vi "HFRR ADV v016 new software.vi"() -> ()   [LabVIEW 2025] (continued)
                        n2565 = local write "EVENT LOG"(w3581) -> ()
                      }
                      frame #28 {
                        n2566 = Wait (ms)(milliseconds to wait=u32 50) -> ()  [unwired: 1 out]
                      }
                      frame #29 {
                        n2567 = local read "Set Rh"() -> (w3585:dbl)
                        n2568 = Number To Fractional String(number=w3585, precision (6)=i16 2) -> (F-format string=w3586:string)  [unwired: 2 in]
                        n2569 = Concatenate Strings("Set Humidity [%RH] :" ("Content"), w3586) -> (w3588:string)
                        n2570 = local read "EVENT LOG"() -> (w3590:string)
                        n2571 = call "Event Log.vi"("Content"=w3588, "EVENT LOG"=w3590) -> ("EVENT LOG"=w3589:string)  [unwired: 8 in, 1 out]
                        n2572 = local write "EVENT LOG"(w3589) -> ()
                      }
                      frame #30 {
                        n2573 = Wait (ms)(milliseconds to wait=u32 50) -> ()  [unwired: 1 out]
                      }
                      frame #31 {
                        n2574 = local read "test time"() -> (w3593:dbl)
                        n2575 = Number To Fractional String(number=w3593, precision (6)=i16 1) -> (F-format string=w3594:string)  [unwired: 2 in]
                        n2576 = Concatenate Strings("Test Duration [mins] :" ("Content"), w3594) -> (w3596:string)
                        n2577 = local read "EVENT LOG"() -> (w3598:string)
                        n2578 = call "Event Log.vi"("Content"=w3596, "EVENT LOG"=w3598) -> ("EVENT LOG"=w3597:string)  [unwired: 8 in, 1 out]
                        n2579 = local write "EVENT LOG"(w3597) -> ()
                      }
                      frame #32 {
                        w3599 = dbl[] [] ("History Data")
                        w3600 = cluster{"y":dbl, dbl, "y":dbl}[] [] ("History Data")
                        w3601 = FALSE ("Visible")
                        n2580 = property on="Stroke ( mm )" class="WFChart (strict)"("History Data"=w3600) -> ()  [unwired: 2 in, 2 out]
                        n2581 = property on="Humidity ( %RH )" class="WFChart (strict)"("History Data"=w3599) -> ()  [unwired: 2 in, 2 out]
                        n2582 = property on="Temperature ( Deg C )" class="WFChart (strict)"("History Data"=w3599) -> ()  [unwired: 2 in, 2 out]
                        n2583 = property on="Electrical Contact Resistance ( % )" class="WFChart (strict)"("History Data"=w3599) -> ()  [unwired: 2 in, 2 out]
                        n2584 = property on="Coefficient of Friction" class="WFChart (strict)"("History Data"=w3599) -> ()  [unwired: 2 in, 2 out]
                        n2585 = property on="Frictional Force ( N )" class="WFChart (strict)"("History Data"=w3599) -> ()  [unwired: 2 in, 2 out]
                        n2586 = property on="Coefficient of Friction" class="WFChart (strict)"("History Data"=w3599) -> ()  [unwired: 2 in, 2 out]
                        n2587 = property on="Frictional Force ( N )" class="WFChart (strict)"("History Data"=w3599) -> ()  [unwired: 2 in, 2 out]
                        n2588 = property on="Electrical Contact Resistance ( % )" class="WFChart (strict)"("History Data"=w3599) -> ()  [unwired: 2 in, 2 out]
                        n2589 = property on="Humidity ( %RH )" class="WFChart (strict)"("History Data"=w3599) -> ()  [unwired: 2 in, 2 out]
                        n2590 = property on="Stroke ( mm )" class="WFChart (strict)"("History Data"=w3600) -> ()  [unwired: 2 in, 2 out]
                        n2591 = property on="Temperature ( Deg C )" class="WFChart (strict)"("History Data"=w3599) -> ()  [unwired: 2 in, 2 out]
                        n2592 = property on="Service Password Log" class="Str"("Visible"=w3601) -> ()  [unwired: 2 in, 2 out]
                        n2593 = property on="Password 3" class="Clust (strict)"("Visible"=w3601) -> ()  [unwired: 2 in, 2 out]
                      }
                    }
                    "TEST FILE NAM,E SAVED" <- TRUE ("TEST FILE NAM,E SAVED")
                  }
                }
              }
            }
          }
        }
        n2594 = case shown="True" w2898 {
          frame False {
            n2595 = local write "tfalg"(0.0 ("tfalg")) -> ()
          }
          frame True {
            n2596 = local read "tfalg"() -> (w3043:dbl)
            n2597 = Equal?(x=w3043, y=0.0) -> (x = y?=w3044:bool)
            n2598 = case shown="True" w3044 {
              frame False {
              }
              frame True {
                n2599 = local read "Total No. of Tests"() -> (w3047:dbl)
                n2600 = local write "tfalg"(1.0 ("tfalg")) -> ()
                n2601 = local write "acq 2"(FALSE ("acq 2")) -> ()
                n2602 = Wait (ms)(milliseconds to wait=u32 200) -> ()  [unwired: 1 out]
                n2603 = Increment(x=w3047) -> (x+1=w3046:dbl)
                n2604 = local write "Total No. of Tests"(w3046) -> ()
              }
            }
          }
        }
        n2605 = local write "Test \nStatus"(w2904) -> ()
        n2606 = local write "Save"(w2904) -> ()
        n2607 = local read "Main Tab"() -> (w2861:T2)
        n2608 = case shown="True" w2885 {
          tunnel: [FALSE ("RUN") TRUE ("RUN")] -> w2884
          tunnel: [_ 1] -> w2877
          frame False {
          }
          frame True {
          }
        }
        n2609 = In Range and Coerce(upper limit=w2892, x=w2865, lower limit=w2891) -> (In Range?=w2883:bool)  [unwired: 1 out]
        n2610 = In Range and Coerce(upper limit=w2889, x=w2864, lower limit=w2890) -> (In Range?=w2881:bool)  [unwired: 1 out]
        n2611 = case shown="True" w2897 {
          frame False {
            n2612 = local read "Rt 3"() -> (w3025:bool)
            n2613 = case shown="True" w3025 {
              frame False {
              }
              frame True {
                n2614 = local write "Rt 3"(FALSE ("Rt 3")) -> ()
                n2615 = local write "Json End Flg"(TRUE ("Upld AR 2")) -> ()
              }
            }
            "Rt" <- TRUE ("Rt")
            "Rt 2" <- FALSE ("Rt")
          }
          frame True {
            n2616 = local read "Rt"() -> (w3032:bool)
            n2617 = local write "Rt 2"(TRUE ("Rt 2")) -> ()
            n2618 = case shown="True" w3032 {
              frame False {
              }
              frame True {
                w3033 = TRUE ("Upld AR 2")
                n2619 = local write "Rt"(FALSE ("Rt")) -> ()
                n2620 = local write "Upld AR"(w3033) -> ()
                n2621 = local write "Json St Flg"(w3033) -> ()
              }
            }
            "Rt 3" <- TRUE ("Rt 3")
          }
        }
        n2622 = case shown="True" w2883 {
          tunnel: [FALSE ("RUN") TRUE ("RUN")] -> w2882
          tunnel: [_ 2] -> w2876
          frame False {
          }
          frame True {
          }
        }
        n2623 = case shown="True" w2881 {
          tunnel: [FALSE ("RUN") TRUE ("RUN")] -> w2880
          tunnel: [_ 3] -> w2875
          frame False {
          }
          frame True {
          }
        }
        n2624 = case shown="\"Acquire\"" w2861 {
          tunnel: w2863 -> [_ w3094]
          frame Default {
            w3093 = 0.0 ("output")
            n2625 = local write "PID-out"(w3093) -> ()
            n2626 = local write "Frequency ( Hz )"(w3093) -> ()
          }
          frame "Acquire" {
            n2627 = stacked-sequence {
              frame #0 {
                n2628 = local read "Auto Start Test"() -> (w3096:bool)
                n2629 = case shown="True" w3096 {
                  tunnel: "RUN" -> [w3117 w3120]
                  tunnel: [w3117 w3119] -> w3097
                  frame False {
                  }
                  frame True {
                    n2630 = local read "Auto Start Temp"() -> (w3118:bool)
                    n2631 = Or(x=w3120, y=w3118) -> (x .or. y?=w3119:bool)
                  }
                }
                n2632 = local read "clk"() -> (w3116:dbl)
                n2633 = local read "Save"() -> (w3112:bool)
                n2634 = Equal?(x=w3116, y=0.0) -> (x = y?=w3113:bool)
                n2635 = And(x=w3113, y=w3112) -> (x .and. y?=w3114:bool)
                n2636 = Not(x="Engage") -> (.not. x?=w3103:bool)
                n2637 = case shown="False" w3097 {
                  tunnel: [0.0 w3143] -> w3099
                  frame False {
                    (unwired) TRUE ("Visible")
                    n2638 = local read "Auto Start Test"() -> (w3124:bool)
                    n2639 = local write "Start Time"(TRUE ("Start Time")) -> ()
                    n2640 = property on="Stroke 2" class="DigNum (strict)"("Visible"=FALSE) -> ()  [unwired: 2 in, 2 out]
                    n2641 = case shown="False" w3124 {
                      frame False {
                        n2642 = property on="Heater Button" class="Bool (strict)"("DisabledEnum"=T18."Enabled" ("Disabled")) -> ()  [unwired: 2 in, 2 out]
                        n2643 = property on="Humidity" class="Bool (strict)"("DisabledEnum"=T18."Enabled" ("Disabled")) -> ()  [unwired: 2 in, 2 out]
                      }
                      frame True {
                      }
                    }
                    n2644 = case shown="False" "TestCompFlg" {
                      frame False {
                        n2645 = local read "StartFlg"() -> (w3132:bool)
                        n2646 = case shown="True" w3132 {
                          frame False {
                          }
                          frame True {
                            n2647 = stacked-sequence {
                              frame #0 {
                                n2648 = local read "EVENT LOG"() -> (w3136:string)
                                n2649 = call "Event Log.vi"("Content"="Test was interrupted", "EVENT LOG"=w3136) -> ("EVENT LOG"=w3137:string)  [unwired: 8 in, 1 out]
                                n2650 = local write "EVENT LOG"(w3137) -> ()
                                n2651 = property on="RUN" class="Bool (strict)"("Visible"=TRUE) -> ()  [unwired: 2 in, 2 out]
                                n2652 = property on="Auto Start Test" class="Bool (strict)"("Visible"=TRUE) -> ()  [unwired: 2 in, 2 out]
                              }
                              frame #1 {
                                w3139 = FALSE ("StartFlg")
                                n2653 = property on="Heater Button" class="Bool (strict)"("Val(Sgnl)"=FALSE ("Value (Signaling)")) -> ()  [unwired: 2 in, 2 out]
                                n2654 = local write "Heater Button"(w3139) -> ()
                                n2655 = local write "StartFlg"(w3139) -> ()
                                n2656 = local write "Humidity"(w3139) -> ()
                              }
                              frame #2 {
                                n2657 = local write "Command"("VC;0" ("Command")) -> ()
                              }
                              frame #3 {
                                n2658 = Wait (ms)(milliseconds to wait=u32 1500) -> ()  [unwired: 1 out]
                              }
                              frame #4 {
                                n2659 = local write "Command"("HE;0" ("Command")) -> ()
                              }
                            }
                          }
                        }
                      }
                      frame True {
                      }
                    }
                    n2660 = local write "String 14"("Test will autostart once parameters reach the set value." ("String 14")) -> ()
                  }
                  frame True {
                    (unwired) FALSE ("Visible")
                    n2661 = property on="Stroke 2" class="DigNum (strict)"("Visible"=TRUE) -> ()  [unwired: 2 in, 2 out]
                    n2662 = property on="STOP 2" class="Bool (strict)"("Disabled"=u8 2) -> ()  [unwired: 2 in, 2 out]
                    n2663 = local write "String 14"(" Running....." ("String 14")) -> ()
                    n2664 = property on="Heater Button" class="Bool (strict)"("DisabledEnum"=T18."Disabled and Grayed Out" ("Disabled")) -> ()  [unwired: 2 in, 2 out]
                    n2665 = property on="Humidity" class="Bool (strict)"("DisabledEnum"=T18."Disabled and Grayed Out" ("Disabled")) -> ()  [unwired: 2 in, 2 out]
                    n2666 = case shown="True" "Start Time" {
                      selector: "Start Time" -> [_ w3162]
                      frame False {
                      }
                      frame True {
                        n2667 = Not(x=w3162) -> (.not. x?=w3161:bool)
                        n2668 = local write "Start Time"(w3161) -> ()
                        n2669 = local read "EVENT LOG"() -> (w3163:string)
                        n2670 = call "Event Log.vi"("Content"="Test in progress", "EVENT LOG"=w3163) -> ("EVENT LOG"=w3165:string)  [unwired: 8 in, 1 out]
                        n2671 = local write "EVENT LOG"(w3165) -> ()
                      }
                    }
                    n2672 = disable-structure shown="Enabled" {
                      disable-tunnel: [w3154 w3160] -> w3143
                      frame Disabled {
                        n2673 = local read "Set Hz"() -> (w3157:dbl)
                        n2674 = call <vilib>:"Uniform White Noise Waveform.vi"() -> ("signal out"=w3156:waveform(dbl))  [unwired: 10 in, 1 out]
                        n2675 = Random Number (0-1)() -> (number: 0 to 1=w3153:dbl)
                        n2676 = Add(x=w3157, y=w3156) -> (x+y=w3155:waveform(dbl))
                        n2677 = Multiply(x=ext 0.01 ("y"), y=w3153) -> (x*y=w3151:ext)
                        n2678 = Multiply(x=w3155, y=w3151) -> (x*y=w3154:waveform(ext))
                      }
                      frame Enabled {
                        n2679 = call-poly <vilib>:"Random Number (Range).vi"("lower bound (0)"=49.89, "upper bound (100)"=50.8) -> ("number"=w3160:dbl)  [unwired: 9 in]
                      }
                    }
                    "StartFlg" <- TRUE ("StartFlg")
                  }
                }
                n2680 = case shown="True" w3114 {
                  frame False {
                  }
                  frame True {
                    n2681 = local write "clk"(10.0 ("clk")) -> ()
                    n2682 = Get Date/Time In Seconds() -> (seconds since 1Jan1904=w3168:timestamp)
                    n2683 = To Double Precision Float(number=w3168) -> (double precision float=w3166:dbl)
                    n2684 = local write "acq timer"(w3166) -> ()
                    n2685 = local write "act save time"(w3166) -> ()
                  }
                }
                n2686 = call "Elapsed Time"("Time Target (s)"="Countdown", "Reset"=w3103) -> ("Elapsed Time (s)"=w3108:dbl, "Time has Elapsed"=w3106:bool)  [unwired: 10 in, 6 out]
                "Countdown 2" <- w3108
                n2687 = Subtract(x=w3108, y=2.0) -> (x-y=w3111:dbl)
                n2688 = Less?(x=w3111, y="Countdown") -> (x < y?=w3109:bool)
                n2689 = And(x=w3109, y=w3106) -> (x .and. y?=w3105:bool)
                n2690 = case shown="True" w3105 {
                  frame False {
                  }
                  frame True {
                    (unwired) dbl[] [] ("History Data")
                    n2691 = local write "Engage"(FALSE ("Engage")) -> ()
                    n2692 = local write "RUN"(TRUE ("RUN")) -> ()
                    n2693 = local read "Humidity ( %RH )"() -> (→"Rh Before":dbl)
                  }
                }
                n2694 = local read "Test \nStatus"() -> (w3101:bool)
                n2695 = Select(t=w3099, s=w3101, f=0.0) -> (s? t:f=w3100:dbl)
                n2696 = local write "Frequency ( Hz )"(w3100) -> ()
              }
              frame #1 {
                w3191 = 1000000.0 ("x")
                # "HC;1/0\nST;VALUE"
                # "Elapsed time\ncof\nstroke\nAir temp\nTemp\nHumidity"
                # "acq timer\n\nact save time"
                # "convert to microseconds"
                n2697 = local read "COUNT"() -> (w3174:i32)
                n2698 = local read "Rate"() -> (w3187:dbl)
                n2699 = Divide(x=w3191, y=w3187) -> (x/y=w3192:dbl)
                n2700 = Greater Or Equal?(x=w3174, y=250) -> (x >= y?=w3173:bool)
                n2701 = Get Date/Time In Seconds() -> (seconds since 1Jan1904=w3194:timestamp)
                n2702 = case shown="True" w3173 {
                  frame False {
                    n2703 = local read "COUNT"() -> (w3195:i32)
                    n2704 = Increment(x=w3195) -> (x+1=w3196:i32)
                    n2705 = local write "COUNT"(w3196) -> ()
                  }
                  frame True {
                    n2706 = local write "COUNT"(0 ("COUNT")) -> ()
                  }
                }
                n2707 = local read "Samplingtime 2"() -> (w3172:dbl)
                n2708 = local read "act save time"() -> (w3189:dbl)
                n2709 = Divide(x=w3192, y=w3191) -> (x/y=w3190:dbl)
                n2710 = To Double Precision Float(number=w3194) -> (double precision float=w3183:dbl)
                n2711 = Add(x=w3189, y=w3172) -> (x+y=w3188:dbl)
                n2712 = local read "acq timer"() -> (w3193:dbl)
                n2713 = local read "COUNT"() -> (w3176:i32)
                n2714 = Greater Or Equal?(x=w3183, y=w3188) -> (x >= y?=w3171:bool)
                n2715 = Multiply(x=w3190, y=w3176) -> (x*y=w3182:dbl)
                n2716 = Subtract(x=w3183, y=w3193) -> (x-y=w3185:dbl)
                n2717 = local read "Save"() -> (w3186:bool)
                n2718 = Add(x=w3185, y=w3182) -> (x+y=w3169:dbl)
                "Elapsed time 3" <- w3169
                n2719 = And(x=w3171, y=w3186) -> (x .and. y?=w3184:bool)
                n2720 = Divide(x=w3169, y=60.0) -> (x/y=w3180:dbl)
                n2721 = local read "Test \nStatus"() -> (w3170:bool)
                n2722 = local read "clk"() -> (w3177:dbl)
                n2723 = Equal?(x=w3177, y=10.0) -> (x = y?=w3179:bool)
                n2724 = case shown="True" w3184 {
                  tunnel: w3183 -> [_ w3307]
                  tunnel: [FALSE ("Boolean 2") TRUE ("Boolean 2")] -> _
                  frame False {
                  }
                  frame True {
                    w3261 = ";" ("Substring")
                    # "Pid out/\nFreq response value"
                    n2725 = local write "act save time"(w3307) -> ()
                    n2726 = local read "FILE"() -> (w3255:string)
                    n2727 = call "file check.vi"("file name in"=w3255) -> ("error out"=w3258:errorcluster, "file name out"=w3253:string)  [unwired: 9 in]
                    n2728 = local read "LVDT STROKE"() -> (w3250:dbl)
                    n2729 = local read "Add up Stroke"() -> (w3248:dbl)
                    n2730 = call "FILE PATH CREATION.vi"("error in"=w3258, "FILE NAME :"=w3253) -> ("FILE OUT"=w3256:path)  [unwired: 8 in, 1 out]
                    n2731 = Concatenate Strings(w3253, ".dgf" ("Substring")) -> (w3257:string)
                    n2732 = Subtract(x=w3250, y=w3248) -> (x-y=w3249:dbl)
                    n2733 = Absolute Value(x=w3249) -> (abs(x)=w3247:dbl)
                    n2734 = local read "FF 2"() -> (→"Frictional Force ( N )" →"Frictional Force ( N )":dbl)
                    n2735 = Build Path(base path=w3256, name or relative path=w3257) -> (appended path=w3252:path)
                    n2736 = local read "COF 2"() -> (w3266:dbl)
                    "cof" <- w3266
                    "Coefficient of Friction" <- w3266
                    "COF 4" <- w3266
                    "Coefficient of Friction" <- w3266
                    n2737 = local read "TEMP"() -> (w3269:dbl)
                    "Temp" <- w3269
                    "Temperature ( Deg C )" <- w3269
                    n2738 = local read "Humidity ( %RH )"() -> (w3268:dbl)
                    "Humidity ( %RH )" <- w3268
                    "Humidity ( %RH )" <- w3268
                    n2739 = local read "Frequency ( Hz )"() -> (w3275:dbl)
                    n2740 = call <vilib>:"Mean PtByPt.vi"("x"=w3247, "sample length"="STROKE FILTER") -> ("mean"=w3246:dbl)  [unwired: 2 in, 1 out]
                    n2741 = local read "Elapsed time"() -> (w3300:dbl)
                    n2742 = local read "AIR TEMP"() -> (w3273:dbl)
                    n2743 = local read "PID-out"() -> (w3278:dbl)
                    n2744 = local write "Temperature ( Deg C )"(w3269) -> ()
                    n2745 = Number To Fractional String(number=w3246, width (-)=i16 9 ("precision (6)"), precision (6)=i16 6) -> (F-format string=w3293:string)  [unwired: 1 in]
                    n2746 = Number To Fractional String(number=w3273, width (-)=i16 9 ("precision (6)"), precision (6)=i16 3) -> (F-format string=w3292:string)  [unwired: 1 in]
                    n2747 = Number To Fractional String(number=w3269, width (-)=i16 9 ("precision (6)"), precision (6)=i16 3) -> (F-format string=w3289:string)  [unwired: 1 in]
                    n2748 = Number To Fractional String(number=w3268, width (-)=i16 9 ("precision (6)"), precision (6)=i16 3) -> (F-format string=w3286:string)  [unwired: 1 in]
                    n2749 = Number To Fractional String(number=0.0, width (-)=i16 9 ("precision (6)"), precision (6)=i16 3) -> (F-format string=w3283:string)  [unwired: 1 in]
                    n2750 = Number To Fractional String(number=w3278, width (-)=i16 9 ("precision (6)"), precision (6)=i16 3) -> (F-format string=w3279:string)  [unwired: 1 in]
                    n2751 = Number To Fractional String(number=w3275, width (-)=i16 9 ("precision (6)"), precision (6)=i16 3) -> (F-format string=w3274:string)  [unwired: 1 in]
                    n2752 = Number To Fractional String(number=w3266, width (-)=i16 9 ("precision (6)"), precision (6)=i16 6) -> (F-format string=w3301:string)  [unwired: 1 in]
                    n2753 = Number To Fractional String(number=w3300, width (-)=i16 14 ("precision (6)"), precision (6)=i16 3) -> (F-format string=w3302:string)  [unwired: 1 in]
                    n2754 = Bundle("y"=1.02, "mean"=w3246, "y"=0.98) -> (w3267:cluster{"y":dbl, "mean":dbl, "y":dbl})  [unwired: 1 in]
                    n2755 = Number To Fractional String(number="Ambient Humidity :", width (-)=i16 9 ("precision (6)"), precision (6)=i16 6) -> (F-format string=w3259:string)  [unwired: 1 in]
                    n2756 = local read "RUN"() -> (w3265:bool)
                    n2757 = case shown="True" w3265 {
                      tunnel: w3267 -> [_ w3312]
                      tunnel: w3246 -> [_ w3311]
                      tunnel: w3246 -> [_ w3309]
                      tunnel: w3246 -> [_ w3310]
                      frame False {
                      }
                      frame True {
                        "Stroke ( mm )" <- w3312
                        "Stroke ( mm )" <- w3312
                        "Stroke 4" <- w3311
                        "Stroke 3" <- w3309
                        "Stroke 2" <- w3310
                        "measured_stroke" <- w3309
                      }
                    }
                    n2758 = Concatenate Strings(w3302, w3261, w3301, w3261, w3293, w3261, w3292, w3261, w3289, w3261, w3286, w3261, w3283, w3261, w3279, w3261, w3274, w3261, w3259, "\r") -> (w3299:string)
                    n2759 = call <vilib>:"Write Characters To File.vi"("append to file? (new file:F)"=TRUE, "character string"=w3299, "file path (dialog if empty)"=w3252) -> ()  [unwired: 2 in, 1 out]
                    "refresh flag" <- TRUE ("refresh flag")
                  }
                }
                n2760 = case shown="True" w3170 {
                  tunnel: w3180 -> [_ w3206]
                  tunnel: w3185 -> [_ w3216]
                  tunnel: [0.0 w3212] -> _
                  tunnel: w3179 -> [_ w3211]
                  tunnel: [0.0 w3210] -> _
                  tunnel: w3169 -> [_ w3210]
                  tunnel: w3183 -> [w3199 _]
                  frame False {
                    n2761 = local write "acq timer"(w3199) -> ()
                    n2762 = local write "Test Duration Status"(0.0 ("Test Duration Status")) -> ()
                  }
                  frame True {
                    n2763 = local read "Set Hz"() -> (w3213:dbl)
                    n2764 = local write "Elapsed time"(w3206) -> ()
                    n2765 = local read "test time"() -> (w3205:dbl)
                    n2766 = Multiply(x=w3216, y=w3213) -> (x*y=w3215:dbl)
                    n2767 = case shown="False" w3211 {
                      tunnel: w3215 -> [w3217 _]
                      tunnel: [w3217 1.0] -> w3212
                      frame False {
                        n2768 = local write "Cycles elapsed"(w3217) -> ()
                      }
                      frame True {
                      }
                    }
                    n2769 = Greater?(x=w3206, y=w3205) -> (0:w3214:bool)
                    n2770 = Subtract(x=w3205, y=w3206) -> (x-y=w3204:dbl)
                    "time" <- w3204
                    n2771 = Multiply(x=w3204, y=60.0) -> (x*y=w3203:dbl)
                    n2772 = local write "Time Remaining"(w3203) -> ()
                    n2773 = local write "Remaining Time"(w3203) -> ()
                    n2774 = case shown="True" w3214 {
                      frame False {
                      }
                      frame True {
                        n2775 = stacked-sequence {
                          frame #0 {
                            w3222 = T18."Enabled" ("Disabled")
                            w3221 = FALSE ("TEST FILE NAM,E SAVED")
                            w3223 = "" ("FILE")
                            w3224 = TRUE ("Visible")
                            n2776 = local write "Humidity"(FALSE ("Humidity")) -> ()
                            n2777 = local write "RUN"(FALSE ("OK Button 2")) -> ()
                            n2778 = local write "Heater Button"(FALSE ("Heater Button")) -> ()
                            n2779 = local write "Auto Start Test"(FALSE ("Auto Start Test")) -> ()
                            n2780 = local write "TestCompFlg"(TRUE ("StpFlg")) -> ()
                            n2781 = local read "Humidity ( %RH )"() -> (→"Rh After":dbl)
                            n2782 = property on="STOP 2" class="Bool (strict)"("Disabled"=u8 0) -> ()  [unwired: 2 in, 2 out]
                            n2783 = local read "EVENT LOG"() -> (w3229:string)
                            n2784 = call "Event Log.vi"("Content"="Test Completed", "EVENT LOG"=w3229) -> ("EVENT LOG"=w3228:string)  [unwired: 8 in, 1 out]
                            n2785 = property on="RUN" class="Bool (strict)"("Visible"=w3224) -> ()  [unwired: 2 in, 2 out]
                            n2786 = property on="Auto Start Test" class="Bool (strict)"("Visible"=w3224) -> ()  [unwired: 2 in, 2 out]
                            n2787 = local write "Batch Ref Num :"(w3223) -> ()
                            n2788 = local write "FILE"(w3223) -> ()
                            n2789 = local write "EVENT LOG"(w3228) -> ()
                            n2790 = local write "TEST FILE NAM,E SAVED"(w3221) -> ()
                            n2791 = local write "Fuel Discription :"(w3223) -> ()
                            n2792 = local write "START TEMP"(w3221) -> ()
                            n2793 = local write "Remarks :"(w3223) -> ()
                            n2794 = local write "Main Dashboard Buttons"(T1."Imaging" ("Main Dashboard Buttons")) -> ()
                            n2795 = local write "Main Tab"(T2."Adv Scar" ("Main Tab")) -> ()
                            n2796 = property on="FRICVALZ 2" class="Bool (strict)"("DisabledEnum"=w3222) -> ()  [unwired: 2 in, 2 out]
                            n2797 = property on="FRICVALZ 3" class="Bool (strict)"("DisabledEnum"=w3222) -> ()  [unwired: 2 in, 2 out]
                            n2798 = property on="FRICVALZ 4" class="Bool (strict)"("DisabledEnum"=w3222) -> ()  [unwired: 2 in, 2 out]
                          }
                          frame #1 {
                            n2799 = Wait (ms)(milliseconds to wait=u32 1500) -> ()  [unwired: 1 out]
                          }
                          frame #2 {
                            n2800 = local write "Command"("VC;0") -> ()
                          }
                          frame #3 {
                            n2801 = Wait (ms)(milliseconds to wait=u32 1500) -> ()  [unwired: 1 out]
                          }
                          frame #4 {
                            n2802 = local write "Command"("VC;0") -> ()
                          }
                          frame #5 {
                            n2803 = Wait (ms)(milliseconds to wait=u32 1500) -> ()  [unwired: 1 out]
                          }
                          frame #6 {
                            n2804 = local write "Command"("ST;0") -> ()
                          }
                          frame #7 {
                            n2805 = local write "measured_stroke"(0.0 ("measured_stroke")) -> ()
                            n2806 = Wait (ms)(milliseconds to wait=u32 1500) -> ()  [unwired: 1 out]
                          }
                          frame #8 {
                            n2807 = local write "Command"("HE;0") -> ()
                          }
                        }
                      }
                    }
                    n2808 = Divide(x=w3206, y=w3205) -> (x/y=w3209:dbl)
                    n2809 = Multiply(x=w3209, y=100.0) -> (x*y=w3207:dbl)
                    n2810 = local write "Test Duration Status"(w3207) -> ()
                  }
                }
              }
              frame #2 {
                n2811 = case shown="True" "Heater Button" {
                  tunnel: [0.0 ("output") w3335] -> w3313
                  frame False {
                    w3316 = TRUE ("tmpchk")
                    n2812 = local read "TEMP"() -> (w3317:dbl)
                    n2813 = local write "Temp ini"(w3317) -> ()
                    n2814 = local write "Reset 4"(w3316) -> ()
                    n2815 = local write "tmpchk"(w3316) -> ()
                    n2816 = local write "reinit"(TRUE ("reinit")) -> ()
                    n2817 = local write "manual temp log"(TRUE ("manual temp log")) -> ()
                  }
                  frame True {
                    # "Logic to turn off\nthe heater when \ntemp is not rising.\nTime - 60 sec\nDelta t- 5°c"
                    n2818 = local read "Temp ini"() -> (w3324:dbl)
                    n2819 = local read "Auto Start Test"() -> (w3320:bool)
                    n2820 = Less?(x=w3324, y=53.0) -> (x < y?=w3322:bool)
                    n2821 = case shown="False" w3320 {
                      frame False {
                        n2822 = local read "Set Temp"() -> (w3344:dbl)
                        n2823 = local read "TEMP"() -> (w3343:dbl)
                        n2824 = Subtract(x=w3344, y=w3343) -> (x-y=w3342:dbl)
                        n2825 = Absolute Value(x=w3342) -> (abs(x)=w3341:dbl)
                        n2826 = Less?(x=w3341, y=0.5) -> (x < y?=w3339:bool)
                        n2827 = case shown="True" w3339 {
                          tunnel: "manual temp log" -> [_ w3345]
                          frame False {
                          }
                          frame True {
                            n2828 = case shown="True" w3345 {
                              selector: w3345 -> [_ w3346]
                              frame False {
                              }
                              frame True {
                                # "#Event log"
                                n2829 = Not(x=w3346) -> (.not. x?=w3347:bool)
                                n2830 = local write "manual temp log"(w3347) -> ()
                                n2831 = local read "EVENT LOG"() -> (w3350:string)
                                n2832 = call "Event Log.vi"("Content"="Target Temperature reached", "EVENT LOG"=w3350) -> ("EVENT LOG"=w3349:string)  [unwired: 8 in, 1 out]
                                n2833 = local write "EVENT LOG"(w3349) -> ()
                              }
                            }
                          }
                        }
                      }
                      frame True {
                        n2834 = local write "manual temp log"(TRUE ("manual temp log")) -> ()
                      }
                    }
                    n2835 = And(x="tmpchk", y=w3322) -> (x .and. y?=w3325:bool)
                    n2836 = case shown="True" w3325 {
                      frame False {
                      }
                      frame True {
                        n2837 = call "Elapsed Time8"("Time Target (s)"=300.0, "Reset"="Reset 4") -> ("Time has Elapsed"=w3352:bool)  [unwired: 10 in, 7 out]
                        n2838 = flat-sequence {
                          tunnel: w3352 -> [_]
                          frame #0 {
                            n2839 = local write "Reset 4"(FALSE ("Reset 4")) -> ()
                          }
                        }
                        n2840 = case shown="True" w3352 {
                          frame False {
                          }
                          frame True {
                            n2841 = local read "Temp ini"() -> (w3359:dbl)
                            n2842 = Add(x=w3359, y=5.0) -> (x+y=w3357:dbl)
                            n2843 = local read "TEMP"() -> (w3360:dbl)
                            n2844 = Greater?(x=w3360, y=w3357) -> (0:w3358:bool)
                            n2845 = case shown="False" w3358 {
                              frame False {
                                n2846 = local write "Heater Button"(FALSE ("Heater Button")) -> ()
                              }
                              frame True {
                                n2847 = local write "tmpchk"(FALSE ("tmpchk")) -> ()
                              }
                            }
                          }
                        }
                      }
                    }
                    n2848 = local read "Set Temp"() -> (w3333:dbl)
                    n2849 = local read "TEMP"() -> (w3327:dbl)
                    n2850 = call-poly <vilib>:"PID.vi"("reinitialize? (F)"="reinit", "dt (s)"=-1.0, "process variable"=w3327, "setpoint"=w3333) -> ("output"=w3330:dbl)  [unwired: 6 in, 1 out]
                    n2851 = Subtract(x=w3333, y=w3327) -> (x-y=w3334:dbl)
                    n2852 = Add(x=w3333, y=0.5) -> (x+y=w3331:dbl)
                    n2853 = Greater Or Equal?(x=w3327, y=w3331) -> ()  [unwired: 1 out]
                    n2854 = Select(t=0.0, s=FALSE, f=w3330) -> (s? t:f=w3329:dbl)
                    "PID output" <- w3329
                    n2855 = flat-sequence {
                      tunnel: w3329 -> [w3363]
                      tunnel: [w3363] -> w3335
                      frame #0 {
                        n2856 = local write "reinit"(FALSE ("reinit")) -> ()
                      }
                    }
                    n2857 = Bundle(w3334, "output"=w3329, "TEMP"=w3327) -> ()  [unwired: 1 in, 1 out]
                  }
                }
                "PID-out" <- w3313
              }
              frame #3 {
                n2858 = local read "TEMP"() -> (w3365:dbl)
                n2859 = Greater Or Equal?(x=w3365, y="Set Temp 2") -> (x >= y?=w3370:bool)
                n2860 = case shown="True" w3370 {
                  tunnel: [FALSE TRUE] -> w3368
                  frame False {
                  }
                  frame True {
                  }
                }
                "Status 13" <- w3368
                n2861 = And(x=w3368, y="trip1 8") -> (x .and. y?=w3367:bool)
                n2862 = case shown="True" w3367 {
                  frame False {
                    n2863 = local write "Heater Trip Temp"(TRUE ("Heater Trip Temp")) -> ()
                  }
                  frame True {
                    w3373 = FALSE ("OK Button 2")
                    n2864 = case shown="True" "Heater Trip Temp" {
                      selector: "Heater Trip Temp" -> [_ w3375]
                      frame False {
                      }
                      frame True {
                        n2865 = Not(x=w3375) -> (.not. x?=w3374:bool)
                        n2866 = local read "EVENT LOG"() -> (w3378:string)
                        n2867 = local write "Heater Trip Temp"(w3374) -> ()
                        n2868 = call "Event Log.vi"("Content"="Heater Trip", "EVENT LOG"=w3378) -> ("EVENT LOG"=w3377:string)  [unwired: 8 in, 1 out]
                        n2869 = local write "EVENT LOG"(w3377) -> ()
                      }
                    }
                    n2870 = local write "RUN"(w3373) -> ()
                    n2871 = property on="Auto Start Test" class="Bool (strict)"("Value"=w3373) -> ()  [unwired: 2 in, 2 out]
                    n2872 = local write "Heater Button"(w3373) -> ()
                  }
                }
              }
            }
            n2873 = case shown="False" w3094 {
              frame False {
                n2874 = disable-structure shown="Disabled" {
                  frame Disabled {
                    n2875 = stacked-sequence {
                      frame #0 {
                        n2876 = local write "RUN"(FALSE ("OK Button 2")) -> ()
                      }
                      frame #1 {
                      }
                    }
                  }
                  frame Enabled {
                  }
                }
              }
              frame True {
              }
            }
          }
        }
        n2877 = local read "airtempflg"() -> (w2886:bool)
        n2878 = Or(x=w2886, y=w2884) -> (x .or. y?=w2887:bool)
        n2879 = Insert Into Array(array=string[] ["Air Temperature has reached set value,", "Humidity has reached set value,", "Sample Temperaturehas reached set value,", ""], index=0, new element="") -> (w2872:string[])
        n2880 = Build Array(w2877, w2876, w2875) -> (w2873:i32[])
        n2881 = disable-structure shown="Disabled" {
          disable-tunnel: w2887 -> [w2964 _]
          disable-tunnel: w2882 -> [w2963 _]
          disable-tunnel: w2880 -> [w2962 _]
          frame Disabled {
            n2882 = Compound Arithmetic op=AND(w2964, w2963, w2962) -> ()  [unwired: 1 out]
            n2883 = case shown="True" {
              selector: _ -> [_ _]
              frame False {
              }
              frame True {
                w2965 = FALSE ("autostrtflg")
                n2884 = local write "RUN"(TRUE ("RUN")) -> ()
                n2885 = local write "autostrtflg"(w2965) -> ()
                n2886 = local write "autostart"(w2965) -> ()
                n2887 = local write "String 14"(" Running....." ("String 14")) -> ()
              }
            }
          }
          frame Enabled {
          }
        }
        n2888 = for {
          tunnel: w2873 -> [w3015] mode=indexing
          tunnel: w2872 -> [w3014]
          shift-right: [w3011] -> w2871
          shift-left: "" -> [w3013]
          n2889 = Index Array(array=w3014, index=w3015) -> (element=w3012:string)
          n2890 = Concatenate Strings(w3012, w3013) -> (w3011:string)
        }
        n2891 = local write "autostart 2"(w2871) -> ()
        n2892 = local read "Reset Graph"() -> (w2860:bool)
        n2893 = case shown="True" w2860 {
          selector: w2860 -> [_ w2914]
          frame False {
          }
          frame True {
            w2928 = 0.0 ("X Scale.Range:Maximum")
            n2894 = Not(x=w2914) -> (.not. x?=w2913:bool)
            n2895 = local write "Reset Graph"(w2913) -> ()
            n2896 = property on="Electrical Contact Resistance ( % )" class="WFChart (strict)"("XScale.Maximum"=600.0 ("X Scale.Range:Maximum"), "XScale.Minimum"=0.0 ("X Scale.Range:Minimum"), "YScale.Maximum"=100.0 ("Y Scale.Range:Maximum"), "YScale.Minimum"=0.0 ("Y Scale.Range:Minimum")) -> ()  [unwired: 2 in, 2 out]
            n2897 = property on="Frictional Force ( N )" class="WFChart (strict)"("XScale.Maximum"=600.0 ("X Scale.Range:Maximum"), "XScale.Minimum"=0.0 ("X Scale.Range:Minimum"), "YScale.Maximum"=100.0 ("Y Scale.Range:Maximum"), "YScale.Minimum"=0.0 ("Y Scale.Range:Minimum")) -> ()  [unwired: 2 in, 2 out]
            n2898 = property on="Temperature ( Deg C )" class="WFChart (strict)"("XScale.Maximum"=600.0 ("X Scale.Range:Maximum"), "XScale.Minimum"=0.0 ("X Scale.Range:Minimum"), "YScale.Maximum"=100.0 ("Y Scale.Range:Maximum"), "YScale.Minimum"=0.0 ("Y Scale.Range:Minimum")) -> ()  [unwired: 2 in, 2 out]
            n2899 = property on="Humidity ( %RH )" class="WFChart (strict)"("XScale.Maximum"=600.0 ("X Scale.Range:Maximum"), "XScale.Minimum"=0.0 ("X Scale.Range:Minimum"), "YScale.Maximum"=100.0 ("Y Scale.Range:Maximum"), "YScale.Minimum"=0.0 ("Y Scale.Range:Minimum")) -> ()  [unwired: 2 in, 2 out]
            n2900 = property on="Stroke ( mm )" class="WFChart (strict)"("XScale.Maximum"=600.0 ("X Scale.Range:Maximum"), "XScale.Minimum"=0.0 ("X Scale.Range:Minimum"), "YScale.Maximum"=100.0 ("Y Scale.Range:Maximum"), "YScale.Minimum"=0.0 ("Y Scale.Range:Minimum")) -> ()  [unwired: 2 in, 2 out]
            n2901 = property on="Coefficient of Friction" class="WFChart (strict)"("XScale.Maximum"=600.0 ("X Scale.Range:Maximum"), "XScale.Minimum"=0.0 ("X Scale.Range:Minimum"), "YScale.Maximum"=100.0 ("Y Scale.Range:Maximum"), "YScale.Minimum"=0.0 ("Y Scale.Range:Minimum")) -> ()  [unwired: 2 in, 2 out]
            n2902 = property on="Electrical Contact Resistance ( % )" class="WFChart (strict)"("XScale.Minimum"=0.0 ("X Scale.Range:Minimum"), "XScale.Maximum"=600.0 ("X Scale.Range:Maximum"), "YScale.Minimum"=0.0 ("Y Scale.Range:Minimum"), "YScale.Maximum"=100.0 ("Y Scale.Range:Maximum")) -> ()  [unwired: 2 in, 2 out]
            n2903 = property on="Temperature ( Deg C )" class="WFChart (strict)"("XScale.Minimum"=0.0 ("X Scale.Range:Minimum"), "XScale.Maximum"=600.0 ("X Scale.Range:Maximum"), "YScale.Minimum"=0.0 ("Y Scale.Range:Minimum"), "YScale.Maximum"=100.0 ("Y Scale.Range:Maximum")) -> ()  [unwired: 2 in, 2 out]
            n2904 = property on="Coefficient of Friction" class="WFChart (strict)"("XScale.Minimum"=0.0 ("X Scale.Range:Minimum"), "XScale.Maximum"=600.0 ("X Scale.Range:Maximum"), "YScale.Maximum"=1.0 ("X Scale.Range:Minimum"), "YScale.Minimum"=0.0 ("X Scale.Range:Minimum")) -> ()  [unwired: 2 in, 2 out]
            n2905 = property on="Frictional Force ( N )" class="WFChart (strict)"("XScale.Maximum"=600.0 ("X Scale.Range:Maximum"), "XScale.Minimum"=w2928, "YScale.Maximum"=10.0 ("Y Scale.Range:Maximum"), "YScale.Minimum"=w2928) -> ()  [unwired: 2 in, 2 out]
            n2906 = property on="Stroke ( mm )" class="WFChart (strict)"("XScale.Maximum"=600.0 ("X Scale.Range:Maximum"), "XScale.Minimum"=0.0 ("X Scale.Range:Minimum"), "YScale.Maximum"=100.0 ("Y Scale.Range:Maximum"), "YScale.Minimum"=0.0 ("Y Scale.Range:Minimum")) -> ()  [unwired: 2 in, 2 out]
            n2907 = property on="Humidity ( %RH )" class="WFChart (strict)"("XScale.Maximum"=600.0 ("X Scale.Range:Maximum"), "XScale.Minimum"=0.0 ("X Scale.Range:Minimum"), "YScale.Maximum"=100.0 ("Y Scale.Range:Maximum"), "YScale.Minimum"=0.0 ("Y Scale.Range:Minimum")) -> ()  [unwired: 2 in, 2 out]
          }
        }
      }
      frame "Compare Files" {
        # "Elapsed time\ncof\nstroke\nAir temp\nTemp\nHumidity"
        n2908 = case shown="True" "RSTV1 2" {
          frame False {
          }
          frame True {
            n2909 = property on="Humidity ( %RH )" class="XYGraph (strict)"("Y Scale.Display Format:Precision"=u8 0 ("Y Scale.Format & Precision:Precision")) -> ()  [unwired: 2 in, 2 out]
            n2910 = property on="Humidity ( %RH )" class="XYGraph (strict)"("X Scale.Range:Minimum"=0.0, "X Scale.Range:Maximum"=75.0, "Y Scale.Range:Minimum"=48.0, "Y Scale.Range:Maximum"=58.0) -> ()  [unwired: 2 in, 2 out]
          }
        }
        n2911 = case shown="True" "RST CP 2" {
          frame False {
          }
          frame True {
            n2912 = property on="XY Graph 13" class="XYGraph (strict)"("Y Scale.Display Format:Precision"=u8 0 ("Y Scale.Format & Precision:Precision")) -> ()  [unwired: 2 in, 2 out]
            n2913 = property on="XY Graph 13" class="XYGraph (strict)"("X Scale.Range:Minimum"=0.0, "X Scale.Range:Maximum"=75.0, "Y Scale.Range:Minimum"=0.0, "Y Scale.Range:Maximum"=100.0) -> ()  [unwired: 2 in, 2 out]
          }
        }
        n2914 = case shown="True" "RST CP" {
          frame False {
          }
          frame True {
            n2915 = property on="Sample Temperature ( °C )" class="XYGraph (strict)"("Y Scale.Display Format:Precision"=u8 2 ("Y Scale.Format & Precision:Precision")) -> ()  [unwired: 2 in, 2 out]
            n2916 = property on="Sample Temperature ( °C )" class="XYGraph (strict)"("X Scale.Range:Minimum"=0.0, "X Scale.Range:Maximum"=75.0, "Y Scale.Range:Minimum"=58.0, "Y Scale.Range:Maximum"=62.0) -> ()  [unwired: 2 in, 2 out]
          }
        }
        n2917 = case shown="True" "RSTV1 3" {
          frame False {
          }
          frame True {
            n2918 = property on="Air Temperature  ( °C )" class="XYGraph (strict)"("Y Scale.Display Format:Precision"=u8 2 ("Y Scale.Format & Precision:Precision")) -> ()  [unwired: 2 in, 2 out]
            n2919 = property on="Air Temperature  ( °C )" class="XYGraph (strict)"("X Scale.Range:Minimum"=0.0 ("Y Scale.Range:Minimum"), "X Scale.Range:Maximum"=75.0 ("Y Scale.Range:Maximum"), "Y Scale.Range:Minimum"=20.0 ("X Scale.Range:Minimum"), "Y Scale.Range:Maximum"=26.0 ("X Scale.Range:Maximum")) -> ()  [unwired: 2 in, 2 out]
          }
        }
        n2920 = case shown="True" "RSTV1 4" {
          frame False {
          }
          frame True {
            n2921 = property on="Stroke ( mm )" class="XYGraph (strict)"("Y Scale.Display Format:Precision"=u8 2 ("Y Scale.Format & Precision:Precision")) -> ()  [unwired: 2 in, 2 out]
            n2922 = property on="Stroke ( mm )" class="XYGraph (strict)"("X Scale.Range:Minimum"=0.0 ("Y Scale.Range:Maximum"), "X Scale.Range:Maximum"=75.0 ("X Scale.Range:Minimum"), "Y Scale.Range:Minimum"=0.98, "Y Scale.Range:Maximum"=1.02) -> ()  [unwired: 2 in, 2 out]
          }
        }
        n2923 = case shown="True" "rstv2" {
          frame False {
          }
          frame True {
            n2924 = property on="Coefficient Of Friction" class="XYGraph (strict)"("Y Scale.Display Format:Precision"=u8 3 ("Y Scale.Format & Precision:Precision")) -> ()  [unwired: 2 in, 2 out]
            n2925 = property on="Coefficient Of Friction" class="XYGraph (strict)"("X Scale.Range:Minimum"=0.0 ("Y Scale.Range:Maximum"), "X Scale.Range:Maximum"=75.0, "Y Scale.Range:Minimum"=0.0, "Y Scale.Range:Maximum"=1.0 ("X Scale.Range:Minimum")) -> ()  [unwired: 2 in, 2 out]
          }
        }
        n2926 = case shown="True" "RST CP 3" {
          frame False {
          }
          frame True {
            n2927 = property on="Air Temp ( °C ) vs Humidity ( % RH )" class="XYGraph (strict)"("X Scale.Range:Minimum"=18.0, "X Scale.Range:Maximum"=28.0 ("X Scale.Range:Minimum"), "Y Scale.Range:Minimum"=30.0 ("X Scale.Range:Minimum"), "Y Scale.Range:Maximum"=70.0 ("X Scale.Range:Minimum")) -> ()  [unwired: 2 in, 2 out]
          }
        }
        n2928 = case shown="True" "OPEN 1" {
          frame False {
          }
          frame True {
            (unwired) 0  # existing file
            w3654 = "Choose a datalog file to open"  # prompt
            n2929 = local write "OPEN 1"(FALSE ("OPEN 1")) -> ()
            n2930 = String To Path(string="C:\\LAB-IQ\\Data\\") -> (path=w3639:path)
            n2931 = File Dialog(6:"*.dgf" ("pattern"), 7:w3654, 11:w3639) -> (0:w3637:errorcluster, 3:w3645:path)  [unwired: 4 in, 2 out]
            n2932 = Unbundle(w3637) -> ()  [unwired: 3 out]
            n2933 = Strip Path(path=w3645) -> (name=w3644:string)  [unwired: 1 out]
            n2934 = Path To String(path=w3645) -> (string=w3640:string)
            "string1" <- w3640
            n2935 = Match Pattern(string=w3644, regular expression=".dgf") -> (before substring=→"String Control":string)  [unwired: 1 in, 3 out]
            n2936 = Match Pattern(string=w3640, regular expression=".dgf" ("substring (\"\")")) -> (before substring=w3650:string)  [unwired: 1 in, 3 out]
            n2937 = Concatenate Strings(w3650, ".duf" ("Substring")) -> (w3646:string)
            n2938 = String To Path(string=w3646) -> (path=w3651:path)
            n2939 = call <vilib>:"Read Characters From File.vi"("file path (dialog if empty)"=w3651, "start of read offset (chars.:0)"=60 ("start of read offset (chars.: 0)")) -> ("character string"=→"String Control 2":string)  [unwired: 4 in, 3 out]
          }
        }
        n2940 = case shown="True" "OPEN 2" {
          frame False {
          }
          frame True {
            (unwired) 0  # existing file
            w3672 = "Choose a datalog file to open"  # prompt
            n2941 = local write "OPEN 2"(FALSE ("OPEN 1")) -> ()
            n2942 = String To Path(string="C:\\LAB-IQ\\Data\\") -> (path=w3657:path)
            n2943 = File Dialog(6:"*.dgf" ("pattern"), 7:w3672, 11:w3657) -> (0:w3655:errorcluster, 3:w3663:path)  [unwired: 4 in, 2 out]
            n2944 = Unbundle(w3655) -> ()  [unwired: 3 out]
            n2945 = Strip Path(path=w3663) -> (name=w3661:string)  [unwired: 1 out]
            n2946 = Path To String(path=w3663) -> (string=w3658:string)
            "string1 2" <- w3658
            n2947 = Match Pattern(string=w3661, regular expression=".dgf") -> (before substring=→"String Control 3":string)  [unwired: 1 in, 3 out]
            n2948 = Match Pattern(string=w3658, regular expression=".dgf" ("substring (\"\")")) -> (before substring=w3669:string)  [unwired: 1 in, 3 out]
            n2949 = Concatenate Strings(w3669, ".duf" ("Substring")) -> (w3666:string)
            n2950 = String To Path(string=w3666) -> (path=w3664:path)
            n2951 = call <vilib>:"Read Characters From File.vi"("file path (dialog if empty)"=w3664, "start of read offset (chars.:0)"=60 ("start of read offset (chars.: 0)")) -> ("character string"=→"String Control 4":string)  [unwired: 4 in, 3 out]
          }
        }
        n2952 = case shown="True" "OPEN 3" {
          frame False {
          }
          frame True {
            (unwired) 0  # existing file
            w3690 = "Choose a datalog file to open"  # prompt
            n2953 = local write "OPEN 3"(FALSE ("OPEN 1")) -> ()
            n2954 = String To Path(string="C:\\LAB-IQ\\Data\\") -> (path=w3675:path)
            n2955 = File Dialog(6:"*.dgf" ("pattern"), 7:w3690, 11:w3675) -> (0:w3673:errorcluster, 3:w3681:path)  [unwired: 4 in, 2 out]
            n2956 = Unbundle(w3673) -> ()  [unwired: 3 out]
            n2957 = Strip Path(path=w3681) -> (name=w3679:string)  [unwired: 1 out]
            n2958 = Path To String(path=w3681) -> (string=w3676:string)
            "string1 3" <- w3676
            n2959 = Match Pattern(string=w3679, regular expression=".dgf") -> (before substring=→"String Control 5":string)  [unwired: 1 in, 3 out]
            n2960 = Match Pattern(string=w3676, regular expression=".dgf" ("substring (\"\")")) -> (before substring=w3686:string)  [unwired: 1 in, 3 out]
            n2961 = Concatenate Strings(w3686, ".duf" ("Substring")) -> (w3683:string)
            n2962 = String To Path(string=w3683) -> (path=w3687:path)
            n2963 = call <vilib>:"Read Characters From File.vi"("file path (dialog if empty)"=w3687, "start of read offset (chars.:0)"=60 ("start of read offset (chars.: 0)")) -> ("character string"=→"String Control 6":string)  [unwired: 4 in, 3 out]
          }
        }
        n2964 = case shown="True" "OPEN 4" {
          frame False {
          }
          frame True {
            (unwired) 0  # existing file
            w3708 = "Choose a datalog file to open"  # prompt
            n2965 = local write "OPEN 4"(FALSE ("OPEN 1")) -> ()
            n2966 = String To Path(string="C:\\LAB-IQ\\Data\\") -> (path=w3693:path)
            n2967 = File Dialog(6:"*.dgf" ("pattern"), 7:w3708, 11:w3693) -> (0:w3691:errorcluster, 3:w3699:path)  [unwired: 4 in, 2 out]
            n2968 = Unbundle(w3691) -> ()  [unwired: 3 out]
            n2969 = Strip Path(path=w3699) -> (name=w3697:string)  [unwired: 1 out]
            n2970 = Path To String(path=w3699) -> (string=w3694:string)
            "string1 4" <- w3694
            n2971 = Match Pattern(string=w3697, regular expression=".dgf") -> (before substring=→"String Control 7":string)  [unwired: 1 in, 3 out]
            n2972 = Match Pattern(string=w3694, regular expression=".dgf" ("substring (\"\")")) -> (before substring=w3704:string)  [unwired: 1 in, 3 out]
            n2973 = Concatenate Strings(w3704, ".duf" ("Substring")) -> (w3701:string)
            n2974 = String To Path(string=w3701) -> (path=w3705:path)
            n2975 = call <vilib>:"Read Characters From File.vi"("file path (dialog if empty)"=w3705, "start of read offset (chars.:0)"=60 ("start of read offset (chars.: 0)")) -> ("character string"=→"String Control 8":string)  [unwired: 4 in, 3 out]
          }
        }
      }
      frame "About" {
        # "Elapsed time\ncof\nstroke\nmean pos\nTemp\nHumidity"
        n2976 = disable-structure shown="Disabled" {
          frame Disabled {
            n2977 = case shown="True" "Export" {
              frame False {
              }
              frame True {
                w3730 = "                                      " ("string")
                w3732 = "\r"
                (unwired) i16 6 ("width (-)")
                w3809 = "\r"
                w3741 = "\r"
                n2978 = local write "Export"(FALSE ("Export")) -> ()
                n2979 = local read "String 29"() -> (w3778:string)
                n2980 = local read "String 34"() -> (w3766:string)
                n2981 = local read "String 35"() -> (w3761:string)
                n2982 = local read "String 37"() -> (w3757:string)
                n2983 = local read "String 36"() -> (w3754:string)
                n2984 = local read "String 38"() -> (w3751:string)
                n2985 = local read "String 39"() -> (w3748:string)
                n2986 = Match Pattern(string=w3778, regular expression=".dwm") -> (before substring=w3774:string)  [unwired: 1 in, 3 out]
                "before substring" <- w3774
                n2987 = local read "S 38"() -> (w3769:string)
                n2988 = local read "S 39"() -> (w3762:string)
                n2989 = local read "Temperature before test 2"() -> (w3798:dbl)
                n2990 = local read "Temperature after test 2"() -> (w3803:dbl)
                n2991 = local read "Humidity before test 2"() -> (w3784:dbl)
                n2992 = local read "Humidity after test 2"() -> (w3799:dbl)
                n2993 = local read "MWSD 2"() -> (w3795:dbl)
                n2994 = local read "WS1.4 2"() -> (w3811:dbl)
                n2995 = local read "HCF 2"() -> (w3807:dbl)
                n2996 = local read "AVP 2"() -> (w3796:dbl)
                n2997 = Concatenate Strings("1," ("string"), w3769) -> (w3768:string)
                n2998 = Concatenate Strings("2," ("string"), w3766) -> (w3765:string)
                n2999 = Concatenate Strings("3," ("string"), w3762) -> (w3764:string)
                n3000 = Concatenate Strings("4," ("string"), w3761) -> (w3760:string)
                n3001 = Concatenate Strings("5," ("string"), w3757) -> (w3758:string)
                n3002 = Concatenate Strings("6," ("string"), w3754) -> (w3755:string)
                n3003 = Concatenate Strings("7," ("string"), w3751) -> (w3752:string)
                n3004 = Concatenate Strings("8," ("string"), w3748) -> (w3749:string)
                n3005 = local read "Sample ID"() -> (w3816:string)
                n3006 = case shown="\"xlx\"" "Select File Type" {
                  tunnel: w3774 -> [w3819 w3821 w3823]
                  tunnel: [w3817 w3822 w3824] -> w3773
                  frame "xlx" {
                    n3007 = Concatenate Strings(w3819, ".xls" ("string")) -> (w3817:string)
                  }
                  frame "csv" {
                    n3008 = Concatenate Strings(w3821, ".csv" ("string")) -> (w3822:string)
                  }
                  frame "txt" {
                    n3009 = Concatenate Strings(w3823, ".txt" ("string")) -> (w3824:string)
                  }
                }
                n3010 = local read "Test Date"() -> (w3815:string)
                n3011 = local read "String 45"() -> (w3729:string)
                n3012 = local read "String 31"() -> (w3814:string)
                n3013 = local read "String 32"() -> (w3813:string)
                n3014 = local read "TITTLE"() -> (w3737:string)
                n3015 = Number To Fractional String(number=w3784, width (-)=i16 6, precision (6)=i16 2) -> (F-format string=w3783:string)  [unwired: 1 in]
                n3016 = Number To Fractional String(number=w3798, width (-)=i16 6, precision (6)=i16 2) -> (F-format string=w3804:string)  [unwired: 1 in]
                n3017 = Number To Fractional String(number=w3799, width (-)=i16 6, precision (6)=i16 2) -> (F-format string=w3797:string)  [unwired: 1 in]
                n3018 = Number To Fractional String(number=w3803, width (-)=i16 6, precision (6)=i16 2) -> (F-format string=w3802:string)  [unwired: 1 in]
                n3019 = Number To Fractional String(number=w3795, width (-)=i16 6, precision (6)=i16 2) -> (F-format string=w3793:string)  [unwired: 1 in]
                n3020 = Number To Fractional String(number=w3796, width (-)=i16 6, precision (6)=i16 2) -> (F-format string=w3794:string)  [unwired: 1 in]
                n3021 = Number To Fractional String(number=w3807, width (-)=i16 6, precision (6)=i16 2) -> (F-format string=w3808:string)  [unwired: 1 in]
                n3022 = Number To Fractional String(number=w3811, precision (6)=i16 2) -> (F-format string=w3812:string)  [unwired: 2 in]
                n3023 = local read "s.NO"() -> (w3731:string)
                n3024 = Concatenate Strings("=" ("string"), w3737) -> (w3736:string)
                n3025 = Concatenate Strings("S.No," ("string"), "                                       Parameters" ("string")) -> (w3742:string)
                n3026 = Concatenate Strings(w3809, w3768, w3783, w3809, w3765, w3804, w3809, w3764, w3797, w3809, w3760, w3802, w3809, w3758, w3793, w3809, w3755, w3794, w3809, w3752, w3808, w3809, w3749, w3812) -> (w3771:string)
                n3027 = Concatenate Strings(w3741, "," ("string"), w3729, w3731, w3730, w3813, w3816, w3730, w3814, w3815, w3741) -> (w3739:string)
                n3028 = local read "Tested by"() -> (w3745:string)
                n3029 = local read "String 33"() -> (w3746:string)
                n3030 = Concatenate Strings("," ("string"), "                                                                             " ("string")) -> (w3734:string)
                n3031 = Concatenate Strings(w3736, w3732, w3739, w3732, w3742, w3771, w3732, w3734, w3746, w3745) -> (→"export":string)
                n3032 = String To Path(string=w3773) -> (path=w3780:path)
                n3033 = local read "export"() -> (w3775:string)
                n3034 = call <vilib>:"Write Characters To File.vi"("append to file? (new file:F)"=FALSE, "character string"=w3775, "file path (dialog if empty)"=w3780) -> ()  [unwired: 2 in, 1 out]
              }
            }
          }
          frame Enabled {
          }
        }
        n3035 = case shown="True" "OK Button 17" {
          frame False {
          }
          frame True {
            (unwired) 0  # existing file
            w4033 = "Choose a datalog file to open"  # prompt
            n3036 = local write "OK Button 17"(FALSE ("OK Button 17")) -> ()
            n3037 = local read "String"() -> (w4028:string)
            n3038 = String To Path(string=w4028) -> (path=w4029:path)
            n3039 = File Dialog(6:"*.duf" ("pattern"), 7:w4033, 11:w4029) -> (0:w4020:errorcluster, 3:w4039:path)  [unwired: 4 in, 2 out]
            n3040 = Unbundle(w4020) -> ()  [unwired: 3 out]
            n3041 = Open/Create/Replace File "Open File"(file path (use dialog)=w4039) -> (refnum out=w4031:refnum<file>)  [unwired: 5 in, 2 out]
            n3042 = Strip Path(path=w4039) -> (name=w4037:string)  [unwired: 1 out]
            n3043 = Path To String(path=w4039) -> (string=w4022:string)
            n3044 = while {
              tunnel: w4031 -> [w4043]
              i -> [w4040]
              stop <- w4041 continue-if-true
              (unwired) TRUE ("line mode (F)")
              n3045 = Read from Text File "Read File"(file (use dialog)=w4043) -> (text=w4042:string)  [unwired: 3 in, 3 out]
              n3046 = local write "Numeric 16"(w4040) -> ()
              n3047 = String Length(string=w4042) -> (length=w4045:i32)
              n3048 = Greater?(x=w4045, y=1) -> (0:w4041:bool)
            }
            n3049 = local write "String 29"(w4022) -> ()
            n3050 = Search and Replace String(input string=w4022, search string=".duf", replace string=".dgf" ("replace string (\"\")")) -> (result string=→"String Indicator 4":string)  [unwired: 5 in, 3 out]
            n3051 = Match Pattern(string=w4037, regular expression=".dwm") -> (before substring=w4021:string)  [unwired: 1 in, 3 out]
            "String Indicator" <- w4021
            n3052 = Match Pattern(string=w4022, regular expression=".dwm" ("substring (\"\")")) -> (before substring=w4023:string)  [unwired: 1 in, 3 out]
            "String Indicator 3" <- w4023
            n3053 = local write "TITTLE 2"(w4021) -> ()
            n3054 = String To Path(string=w4023) -> (path=w4030:path)
            "path" <- w4030
            n3055 = call <vilib>:"Read Characters From File.vi"("file path (dialog if empty)"=w4030, "start of read offset (chars.:0)"=60 ("start of read offset (chars.: 0)")) -> ("character string"=→"String Indicator 2":string)  [unwired: 4 in, 3 out]
          }
        }
        n3056 = call <vilib>:"Query Available Printers.vi"() -> ("system configured printers"=w3722:string[])  [unwired: 9 in, 2 out]
        "System Configured Printers 2" <- w3722
        n3057 = local read "OK Button 16"() -> (w3719:bool)
        n3058 = case shown="True" "OK Button 16" {
          frame False {
          }
          frame True {
            n3059 = stacked-sequence {
              frame #0 {
                n3060 = local read "Numeric 16"() -> (w4047:i32)
